vi "AIsFIFORT_ECD.vi"(0 "FPGA-VI-Referenz":refnum<k20>, 1 "P2":dbl[](array[numeric]), 2 "P1":dbl[](array[numeric]), 3 "P0":dbl[](array[numeric]), 4 "error in":errorcluster) -> (5 "error out":errorcluster)   [LabVIEW 2017]
uses:
  gvbooleschRT.vi
  <vilib>/Utility/error.llb/Error Cluster From Error Code.vi
  <vilib>/rvi/errors/niLvFpgaAdjustHostInterfaceError.vi
  GVAIs.vi
  <vilib>/rvi/interface/nirviMethod/nirviMethod.xnode
  FPGA Bitfiles/HAGAR-VECD_FPGATarget_FPGA-ProgrammECD_WS++LmW9gGg.lvbitx
  FPGA-Programm_ECD.vi
  <vilib>/rvi/interface/nirviReadWriteControl/nirviReadWriteControl.xnode
  <vilib>/rvi/errors/niLvFpgaMergeErrorWithErrorCode.vi
  <vilib>/FPGAPlugInAG/cRIO-9035/niLvFpga_ReadFifo_cRIO-9035.vi
  NiFpgaLv.dll
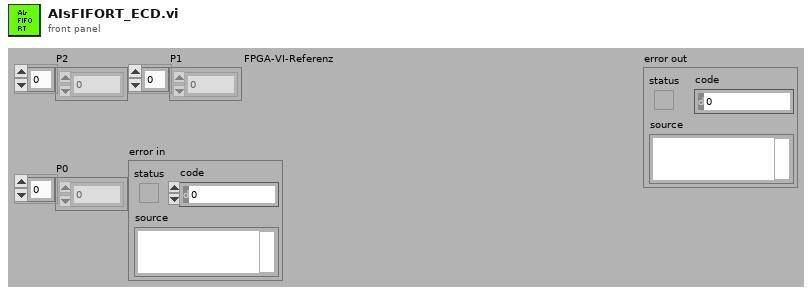
[diagram p1: front panel]
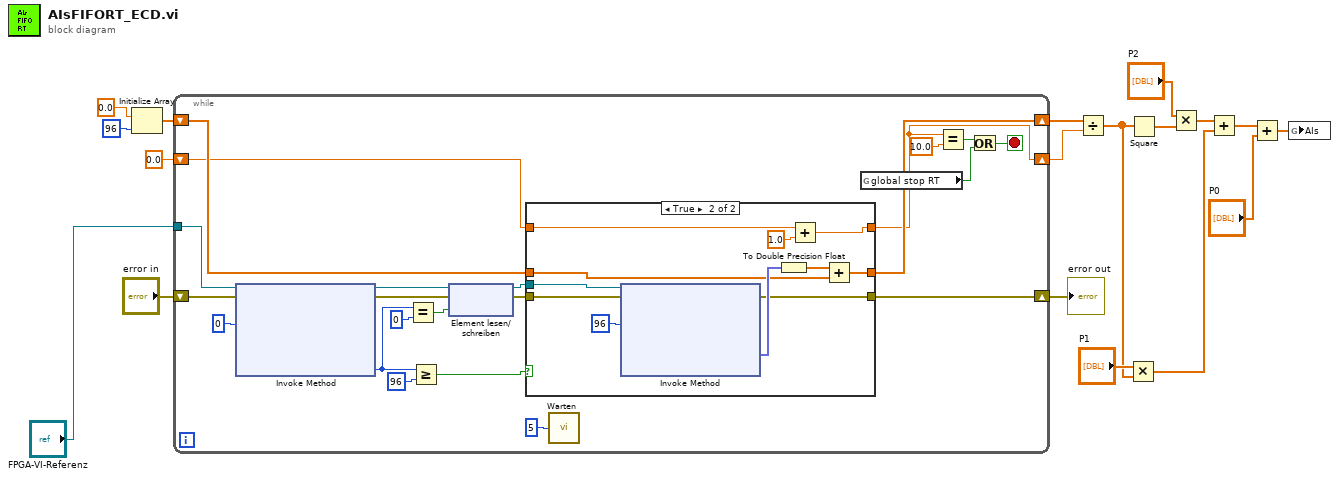
[diagram p0: block diagram]
diagram:
  n1 = Initialize Array(0.0 ("Element"), 96 ("Dimension")) -> (w6:dbl[])
  n2 = while {
    tunnel: "FPGA-VI-Referenz" -> [w40]
    shift-right: [w34] -> w17
    shift-left: w6 -> [w35]
    shift-right: [w32] -> w5
    shift-left: 0.0 -> [w33]
    shift-right: [w19] -> w2
    shift-left: "error in" -> [w22]
    stop <- w25 stop-if-true
    n3 = xnode "Invoke Method"("FPGA-VI-Referenz (Eingang)"=w40, "Fehler (Eingang)"=w22, "Anzahl der Elemente"=u32 0 ("Number of Elements")) -> ("FPGA-VI-Referenz (Ausgang)"=w23:refnum<k20>, "Fehler (Ausgang)"=w21:errorcluster, "Verbleibende Elemente"=w30:u32)  [unwired: 1 in, 1 out]
    n4 = Equal?(x=w30, y=u32 0) -> (x = y?=w28:bool)
    n5 = Greater Or Equal?(x=w30, y=u32 96) -> (x >= y?=w37:bool)
    n6 = xnode "Element lesen/schreiben"("FPGA-VI-Referenz (Eingang)"=w23, "Fehler (Eingang)"=w21, "FIFO leer"=w28) -> ("FPGA-VI-Referenz (Ausgang)"=w24:refnum<k20>, "Fehler (Ausgang)"=w20:errorcluster)
    n7 = case shown="True" w37 {
      tunnel: w24 -> [_ w54]
      tunnel: w35 -> [w43 w50]
      tunnel: [w43 w49] -> w34
      tunnel: w33 -> [w42 w48]
      tunnel: [w42 w46] -> w32
      tunnel: w20 -> [w41 w45]
      tunnel: [w41 w44] -> w19
      frame False {
      }
      frame True {
        n8 = xnode "Invoke Method"("FPGA-VI-Referenz (Eingang)"=w54, "Fehler (Eingang)"=w45, "Anzahl der Elemente"=u32 96 ("Number of Elements")) -> ("Fehler (Ausgang)"=w44:errorcluster, "Daten"=w52:fxp<+/-,26,5>[])  [unwired: 1 in, 2 out]
        n9 = To Double Precision Float(number=w52) -> (double precision float=w51:dbl[])
        n10 = Add(x=w48, y=1.0) -> (x+y=w46:dbl)
        n11 = Add(x=w51, y=w50) -> (x+y=w49:dbl[])
      }
    }
    n12 = call "Warten"("Count(mSec)"=u32 5) -> ()  [unwired: 1 out]
    n13 = global read "gvbooleschRT.vi" "global stop RT"() -> (w27:bool)
    n14 = Equal?(x=w32, y=10.0) -> (x = y?=w26:bool)
    n15 = Or(x=w26, y=w27) -> (x .or. y?=w25:bool)
  }
  "error out" <- w2
  n16 = Divide(x=w17, y=w5) -> (x/y=w13:dbl[])
  n17 = Multiply(x="P1", y=w13) -> (x*y=w11:dbl[])
  n18 = Square(x=w13) -> (x^2=w16:dbl[])
  n19 = Multiply(x="P2", y=w16) -> (x*y=w12:dbl[])
  n20 = Add(x=w12, y=w11) -> (x+y=w10:dbl[])
  n21 = Add(x=w10, y="P0") -> (x+y=w4:dbl[])
  n22 = global write "GVAIs.vi" "AIs"(w4) -> ()
